vi "Draw Tree.vi"(11 "picture":refnum<vi>) -> (3 "2D Picture":picture)   [LabVIEW 2025]
uses:
  <vilib>/picture/picture.llb/imagedata.ctl
  Types/Single Cmd Info.ctl
  Types/Sequencing Tree Node.ctl
  <vilib>/Analysis/NI_AALBase.lvlib
  <vilib>/Analysis/baseanly.llb/Mean (DBL).vi
panel:
  in  "Command Height":dbl=42.0
  in  "Path on Command Branch Height":dbl=53.0
  in  "Default Path Height":dbl=25.0
  in  "Leaf Height":dbl=10.0
  in  "Leaf Circle Radius":i16
  in  "pen":T1={"Width"=3, "Style"=enum."Solid"}
  in  "2D Picture":picture
  in  "Column Gap":dbl=30.0
  in  "Line Thickness":dbl=3.0 format="%#_13g"
  in  "[user-specified font]":T2={"Font Name:"="Bahnschrift", "Size"=15, "Strikeout?"=FALSE, "Italic?"=FALSE, "Underline?"=FALSE, "Outline?"=FALSE, "Shadow?"=FALSE, "Bold?"=FALSE}
  in  "Width Padding":dbl=5.0 format="%#_13g"
  in  "Row Gap":dbl=30.0
  in  "Sequencing Data":T3[](array[typedef])
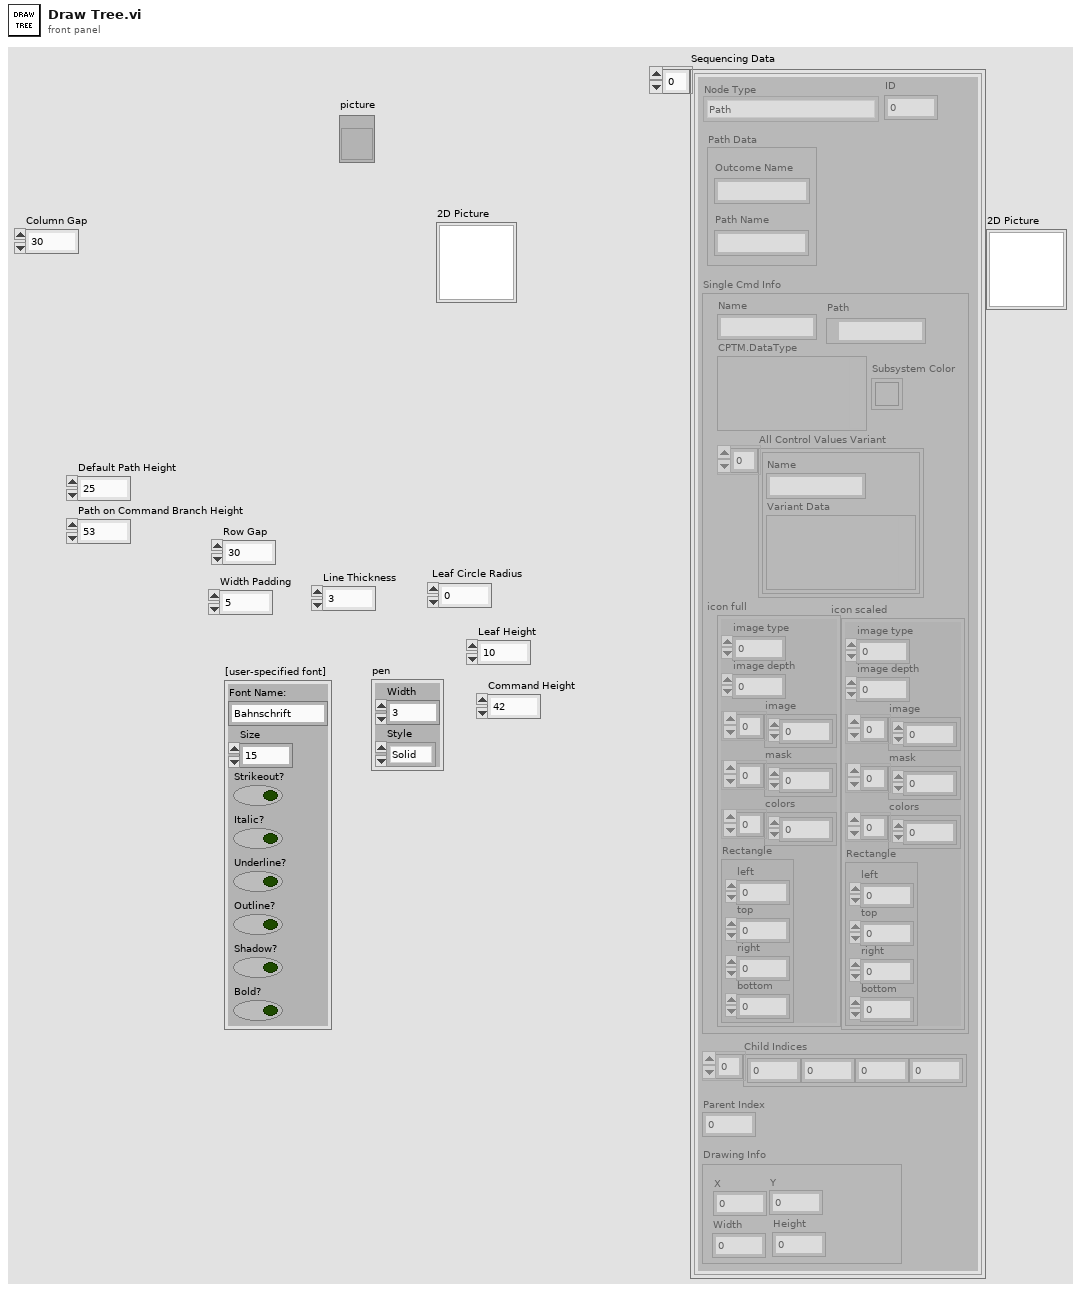
[diagram p1: front panel]
types:
  T1 = cluster{"Width":i16, "Style":enum32{"Solid", "Dash", "Dot", "DashDot", "DashDotDot"}}
  T2 = cluster{"Font Name:":string, "Size":i16, "Strikeout?":bool, "Italic?":bool, "Underline?":bool, "Outline?":bool, "Shadow?":bool, "Bold?":bool}
  T3 = typedef "Sequencing Tree Node.ctl" = cluster{"Node Type":enum16{"Path", "Command", "Leaf"}, "ID":i16, "Path Data":cluster{"Path Name":string, "Outcome Name":string}, "Single Cmd Info":T4, "Child Indices":i32[], "Parent Index":i32, "Drawing Info":cluster{"X":dbl, "Y":dbl, "Width":dbl, "Height":dbl}}
  T4 = typedef "Single Cmd Info.ctl" = cluster{"Name":string, "CPTM.DataType":variant, "All Control Values Variant":cluster{"Name":string, "Variant Data":variant}[], "icon full":T5, "icon scaled":T5, "Path":path, "Subsystem Color":u32}
  T5 = typedef "imagedata.ctl" = cluster{"image type":i32, "image depth":i32, "image":u8[], "mask":u8[], "colors":u32[], "Rectangle":cluster{"left":i16, "top":i16, "right":i16, "bottom":i16}}
  T6 = enum16{"User-specified Font", "Application Font", "System Font", "Dialog Font"}
  T7 = cluster{"Path Name":string, "Outcome Name":string}
  T8 = cluster{"X":dbl, "Y":dbl, "Width":dbl, "Height":dbl}
  T9 = cluster{"left":i16, "top":i16, "right":i16, "bottom":i16}
  T10 = cluster{"[0]":dbl, "[1]":dbl, "[2]":dbl, "[3]":dbl}
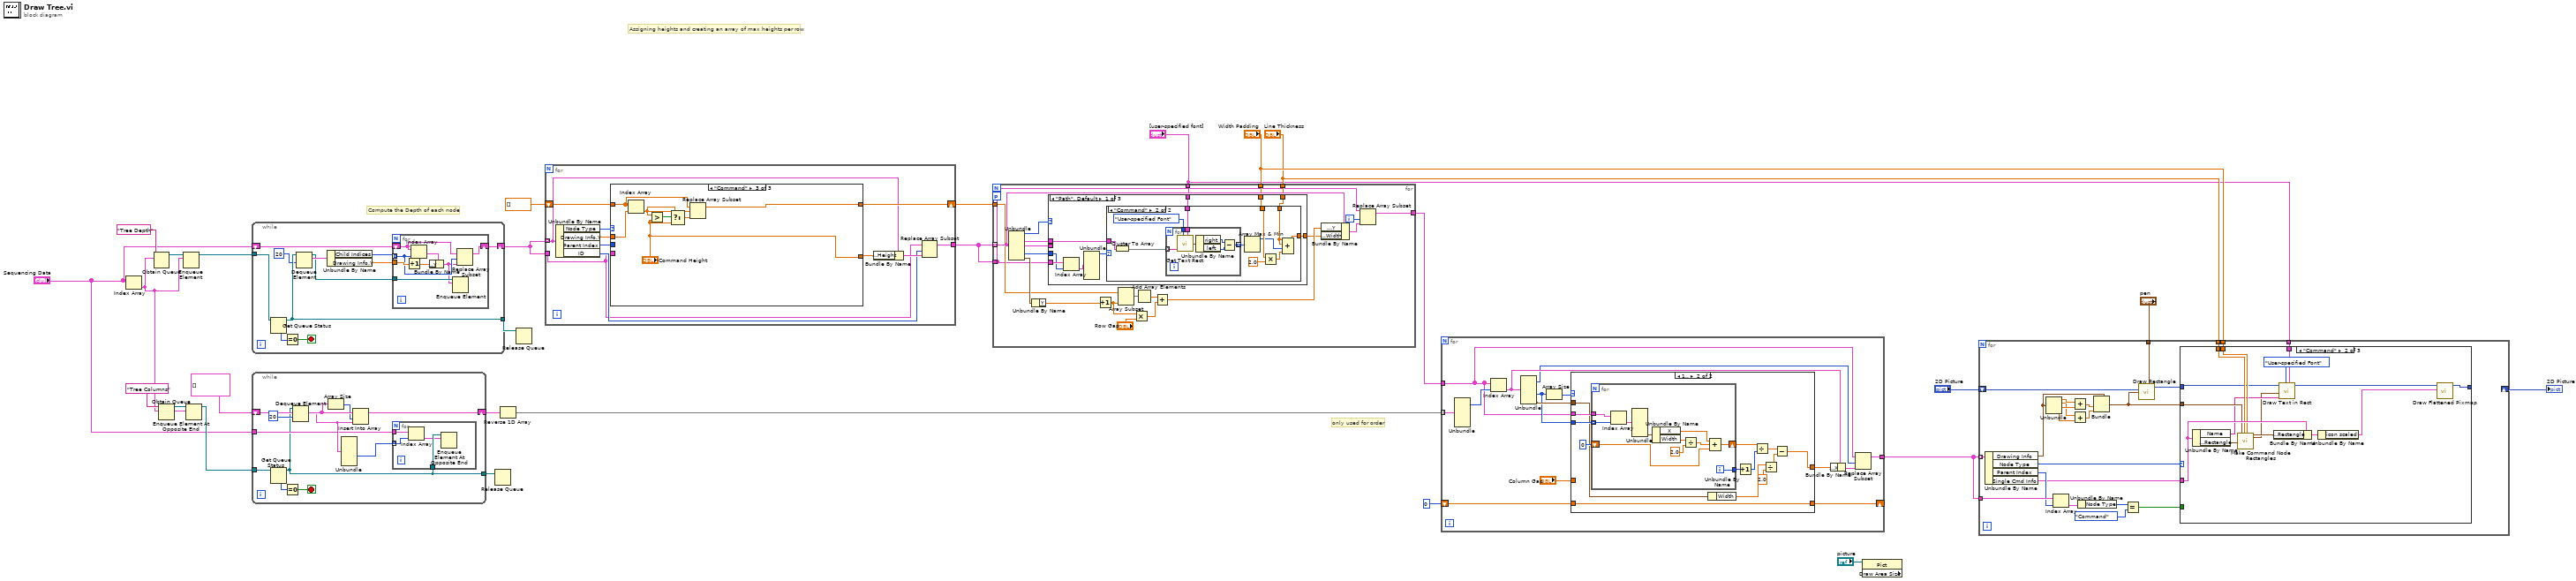
[diagram p0: block diagram]
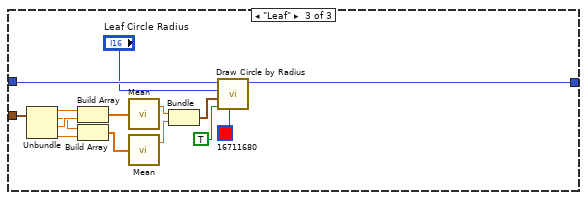
[diagram p3: hidden frame]
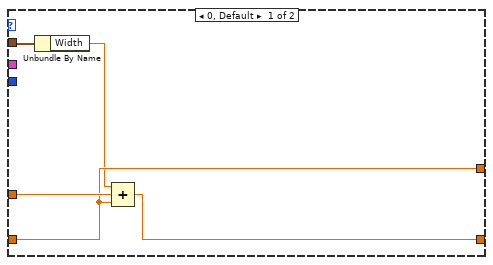
[diagram p4: hidden frame]
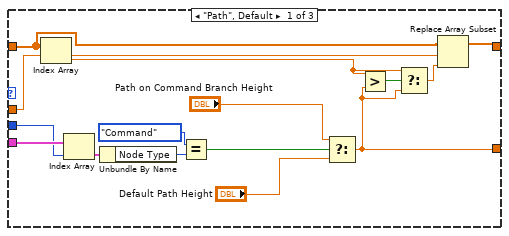
[diagram p5: hidden frame]
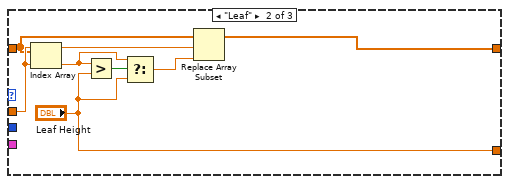
[diagram p6: hidden frame]
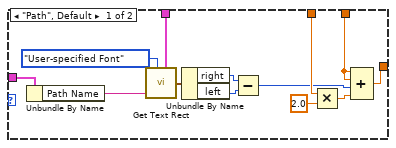
[diagram p7: hidden frame]
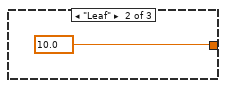
[diagram p8: hidden frame]
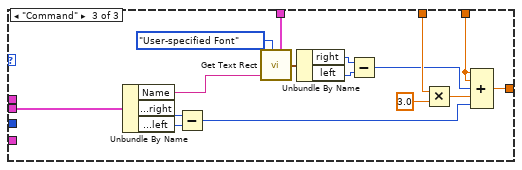
[diagram p9: hidden frame]
diagram:
  # "only used for order"
  # "Assigning heights and creating an array of max heights per row"
  # "Compute the Depth of each node"
  n1 = Index Array(array="Sequencing Data") -> (element=w19:T3)  [unwired: 1 in]
  n2 = Obtain Queue(name (unnamed)="Tree Depth", element data type=w19) -> (queue out=w25:refnum<queue>)  [unwired: 3 in, 2 out]
  n3 = Obtain Queue(name (unnamed)="Tree Columns", element data type=w19) -> (queue out=w21:refnum<queue>)  [unwired: 3 in, 2 out]
  n4 = Enqueue Element(queue=w25, element=w19) -> (queue out=w24:refnum<queue>)  [unwired: 2 in, 2 out]
  n5 = Enqueue Element At Opposite End(queue=w21, element=w19) -> (queue out=w20:refnum<queue>)  [unwired: 2 in, 2 out]
  n6 = while {
    tunnel: w24 -> [w32]
    shift-right: [w34] -> w13
    shift-left: "Sequencing Data" -> [w35]
    tunnel: [w30] -> w22
    stop <- w38 stop-if-true
    n7 = Get Queue Status(queue=w32) -> (queue out=w30:refnum<queue>, # elements in queue=w33:i32)  [unwired: 2 in, 6 out]
    n8 = Equal To 0?(x=w33) -> (x = 0?=w38:bool)
    n9 = Dequeue Element(queue=w30, timeout in ms (-1)=20) -> (queue out=w31:refnum<queue>, element=w37:T3)  [unwired: 1 in, 2 out]
    n10 = Unbundle By Name(w37) -> ("Child Indices"=w36:i32[], "Drawing Info.Y"=w28:dbl)
    n11 = for {
      tunnel: w36 -> [w43] mode=indexing
      tunnel: w28 -> [w46]
      shift-right: [w42] -> w34
      shift-left: w35 -> [w44]
      tunnel: w31 -> [w41]
      n12 = Increment(x=w46) -> (x+1=w39:dbl)
      n13 = Index Array(array=w44, index=w43) -> (element=w45:T3)
      n14 = Bundle By Name(cluster=w45, "Drawing Info.Y"=w39) -> (w40:T3)
      n15 = Enqueue Element(queue=w41, element=w40) -> ()  [unwired: 2 in, 3 out]
      n16 = Replace Array Subset(array=w44, new element=w40, index=w43) -> (w42:T3[])
    }
  }
  n17 = while {
    tunnel: [w48] -> w18
    shift-right: [w51] -> w17
    shift-left: T3[] [] ("Sequencing Data 2") -> [w53]
    tunnel: w20 -> [w55]
    tunnel: "Sequencing Data" -> [w49]
    stop <- w57 stop-if-true
    n18 = Get Queue Status(queue=w55) -> (queue out=w48:refnum<queue>, # elements in queue=w56:i32)  [unwired: 2 in, 6 out]
    n19 = Equal To 0?(x=w56) -> (x = 0?=w57:bool)
    n20 = Dequeue Element(queue=w48, timeout in ms (-1)=20) -> (element=w50:T3)  [unwired: 1 in, 3 out]
    n21 = Array Size(array=w53) -> (size(s)=w52:i32)
    n22 = Unbundle(w50) -> ("Child Indices"=w47:i32[])  [unwired: 6 out]
    n23 = Insert Into Array(array=w53, index=w52, new element=w50) -> (w51:T3[])
    n24 = for {
      tunnel: w47 -> [w60] mode=indexing
      tunnel: w49 -> [w61]
      tunnel: w48 -> [w59]
      n25 = Index Array(array=w61, index=w60) -> (element=w58:T3)
      n26 = Enqueue Element At Opposite End(queue=w59, element=w58) -> ()  [unwired: 2 in, 3 out]
    }
  }
  n27 = Release Queue(queue=w18) -> ()  [unwired: 2 in, 3 out]
  n28 = Reverse 1D Array(array=w17) -> (reversed array=w10:T3[])
  n29 = Release Queue(queue=w22) -> ()  [unwired: 2 in, 3 out]
  n30 = for {
    tunnel: w13 -> [w67] mode=indexing
    shift-right: [w69] -> w12
    shift-left: dbl[] [] -> [w70]
    tunnel: w13 -> [w63]
    tunnel: [w62] -> w11
    n31 = Unbundle By Name(w67) -> ("Node Type"=w72:enum16{"Path", "Command", "Leaf"}, "Drawing Info.Y"=w71:dbl, "Parent Index"=w68:i32, "ID"=w64:i16)
    n32 = case shown="\"Command\"" w72 {
      tunnel: w71 -> [w80 w91 w98]
      tunnel: w70 -> [w81 w90 w97]
      tunnel: [w79 w89 w96] -> w69
      tunnel: w63 -> [w87 _ _]
      tunnel: w68 -> [w86 _ _]
      tunnel: [w77 "Leaf Height" "Command Height"] -> w66
      frame "Path", Default {
        n33 = Index Array(array=w81, index=w80) -> (element=w83:dbl)
        n34 = Index Array(array=w87, index=w86) -> (element=w76:T3)
        n35 = Unbundle By Name(w76) -> ("Node Type"=w75:enum16{"Path", "Command", "Leaf"})
        n36 = Equal?(x=enum16{"Path", "Command", "Leaf"}."Command", y=w75) -> (x = y?=w85:bool)
        n37 = Select(t="Path on Command Branch Height", s=w85, f="Default Path Height") -> (s? t:f=w77:dbl)
        n38 = Greater?(x=w83, y=w77) -> (0:w84:bool)
        n39 = Select(t=w83, s=w84, f=w77) -> (s? t:f=w82:dbl)
        n40 = Replace Array Subset(array=w81, new element=w82, index=w80) -> (w79:dbl[])
      }
      frame "Leaf" {
        n41 = Index Array(array=w90, index=w91) -> (element=w93:dbl)
        n42 = Greater?(x=w93, y="Leaf Height") -> (0:w94:bool)
        n43 = Select(t=w93, s=w94, f="Leaf Height") -> (s? t:f=w92:dbl)
        n44 = Replace Array Subset(array=w90, new element=w92, index=w91) -> (w89:dbl[])
      }
      frame "Command" {
        n45 = Index Array(array=w97, index=w98) -> (element=w100:dbl)
        n46 = Greater?(x=w100, y="Command Height") -> (0:w101:bool)
        n47 = Select(t=w100, s=w101, f="Command Height") -> (s? t:f=w99:dbl)
        n48 = Replace Array Subset(array=w97, new element=w99, index=w98) -> (w96:dbl[])
      }
    }
    n49 = Bundle By Name(cluster=w67, "Drawing Info.Height"=w66) -> (w65:T3)
    n50 = Replace Array Subset(array=w63, new element=w65, index=w64) -> (w62:T3[])
  }
  n51 = for {
    tunnel: w11 -> [w122] mode=indexing
    tunnel: w12 -> [w120]
    workers-P: _ -> [_]
    tunnel: "Width Padding" -> [w111]
    tunnel: "[user-specified font]" -> [w110]
    tunnel: "Line Thickness" -> [w108]
    tunnel: w11 -> [w105]
    tunnel: [w102] -> w9
    i -> [w104]
    n52 = Unbundle(w122) -> ("Node Type"=w123:enum16{"Path", "Command", "Leaf"}, "Path Data"=w106:T7, "Single Cmd Info"=w112:T4, "Parent Index"=w107:i32, "Drawing Info"=w121:T8)  [unwired: 2 out]
    n53 = Unbundle By Name(w121) -> ("Y"=w117:dbl)
    n54 = case shown="\"Path\", Default" w123 {
      tunnel: w112 -> [_ _ w180]
      tunnel: w111 -> [w128 _ w176]
      tunnel: w110 -> [w127 _ w175]
      tunnel: [w124 w164 w169] -> w109
      tunnel: w108 -> [w126 _ w165]
      tunnel: w105 -> [w132 _ _]
      tunnel: w107 -> [w131 _ _]
      tunnel: w106 -> [w125 _ _]
      frame "Path", Default {
        n55 = Index Array(array=w132, index=w131) -> (element=w130:T3)
        n56 = Unbundle(w130) -> ("Node Type"=w129:enum16{"Path", "Command", "Leaf"})  [unwired: 6 out]
        n57 = case shown="\"Command\"" w129 {
          tunnel: w128 -> [w140 w153]
          tunnel: w127 -> [w139 w152]
          tunnel: w126 -> [w136 w151]
          tunnel: w125 -> [w138 w150]
          tunnel: [w133 w146] -> w124
          frame "Path", Default {
            n58 = Unbundle By Name(w138) -> ("Path Name"=w137:string)
            n59 = call <vilib>:"Get Text Rect.vi"("desired font(Application)"=T6."User-specified Font", "text"=w137, "[user-specified font]"=w139) -> ("rect"=w143:T9)  [unwired: 6 in]
            n60 = Unbundle By Name(w143) -> ("right"=w142:i16, "left"=w141:i16)
            n61 = Subtract(x=w142, y=w141) -> (x-y=w135:i16)
            n62 = Multiply(x=w140, y=2.0) -> (x*y=w134:dbl)
            n63 = Compound Arithmetic op=ADD(w136, w136, w135, w134) -> (w133:dbl)
          }
          frame "Command" {
            n64 = Cluster To Array(cluster=w150) -> (array=w149:string[])
            n65 = for {
              tunnel: T6."User-specified Font" ("desired font(Application)") -> [w163]
              tunnel: [w159] -> w148 mode=indexing
              tunnel: w152 -> [w158]
              tunnel: w149 -> [w157] mode=indexing
              n66 = call <vilib>:"Get Text Rect.vi"("desired font(Application)"=w163, "text"=w157, "[user-specified font]"=w158) -> ("rect"=w162:T9)  [unwired: 6 in]
              n67 = Unbundle By Name(w162) -> ("right"=w161:i16, "left"=w160:i16)
              n68 = Subtract(x=w161, y=w160) -> (x-y=w159:i16)
            }
            n69 = Array Max & Min(array=w148) -> (max value=w147:i16)  [unwired: 3 out]
            n70 = Multiply(x=w153, y=2.0) -> (x*y=w154:dbl)
            n71 = Compound Arithmetic op=ADD(w151, w151, w147, w154) -> (w146:dbl)
          }
        }
      }
      frame "Leaf" {
        w164 = 10.0 items=["Leaf"=10.0, "Default Path"=25.0, "Command"=42.0, "Path on Command Branch"=53.0] ("Height")
      }
      frame "Command" {
        n72 = Unbundle By Name(w180) -> ("Name"=w173:string, "icon scaled.Rectangle.right"=w179:i16, "icon scaled.Rectangle.left"=w178:i16)
        n73 = Subtract(x=w179, y=w178) -> (x-y=w168:i16)
        n74 = call <vilib>:"Get Text Rect.vi"("desired font(Application)"=T6."User-specified Font", "text"=w173, "[user-specified font]"=w175) -> ("rect"=w172:T9)  [unwired: 6 in]
        n75 = Unbundle By Name(w172) -> ("right"=w171:i16, "left"=w170:i16)
        n76 = Subtract(x=w171, y=w170) -> (x-y=w166:i16)
        n77 = Multiply(x=w176, y=3.0) -> (x*y=w167:dbl)
        n78 = Compound Arithmetic op=ADD(w165, w165, w166, w167, w168) -> (w169:dbl)
      }
    }
    n79 = Increment(x=w117) -> (x+1=w116:dbl)
    n80 = Array Subset(array=w120, length=w116) -> (w119:dbl[])  [unwired: 1 in]
    n81 = Multiply(x=w116, y="Row Gap") -> (x*y=w114:dbl)
    n82 = Add Array Elements(numeric array=w119) -> (sum=w118:dbl)
    n83 = Add(x=w118, y=w114) -> (x+y=w113:dbl)
    n84 = Bundle By Name(cluster=w122, "Drawing Info.Y"=w113, "Drawing Info.Width"=w109) -> (w103:T3)
    n85 = Replace Array Subset(array=w105, new element=w103, index=w104) -> (w102:T3[])
  }
  n86 = for {
    tunnel: w10 -> [w194] mode=indexing
    tunnel: w9 -> [w183]
    shift-right: [w186] -> _
    shift-left: 0 -> [w191]
    tunnel: [w181] -> w4
    n87 = Unbundle(w194) -> ("ID"=w193:i16)  [unwired: 6 out]
    n88 = Index Array(array=w183, index=w193) -> (element=w190:T3)
    n89 = Unbundle(w190) -> ("ID"=w182:i16, "Child Indices"=w185:i32[], "Drawing Info"=w187:T8)  [unwired: 4 out]
    n90 = Array Size(array=w185) -> (size(s)=w192:i32)
    n91 = case shown="1.." w192 {
      tunnel: w191 -> [w196 w212]
      tunnel: [w196 w200] -> w189
      tunnel: "Column Gap" -> [w197 _]
      tunnel: w187 -> [w199 w202]
      tunnel: [w198 w212] -> w186
      tunnel: w185 -> [_ w211]
      tunnel: w183 -> [_ w210]
      frame 0, Default {
        n92 = Unbundle By Name(w199) -> ("Width"=w195:dbl)
        n93 = Compound Arithmetic op=ADD(w195, w197, w196) -> (w198:dbl)
      }
      frame 1.. {
        n94 = for {
          tunnel: w211 -> [w223] mode=indexing
          tunnel: w210 -> [w222]
          shift-right: [w214] -> w208
          shift-left: 0 -> [w215]
          tunnel: [w213] -> w207
          i -> [w213]
          n95 = Index Array(array=w222, index=w223) -> (element=w221:T3)
          n96 = Unbundle(w221) -> ("Drawing Info"=w220:T8)  [unwired: 6 out]
          n97 = Unbundle By Name(w220) -> ("X"=w217:dbl, "Width"=w219:dbl)
          n98 = Divide(x=w219, y=2.0) -> (x/y=w216:dbl)
          n99 = Compound Arithmetic op=ADD(w217, w216, w215) -> (w214:dbl)
        }
        n100 = Unbundle By Name(w202) -> ("Width"=w201:dbl)
        n101 = Increment(x=w207) -> (x+1=w206:i32)
        n102 = Divide(x=w208, y=w206) -> (x/y=w205:dbl)
        n103 = Divide(x=w201, y=2.0) -> (x/y=w204:dbl)
        n104 = Subtract(x=w205, y=w204) -> (x-y=w200:dbl)
      }
    }
    n105 = Bundle By Name(cluster=w190, "Drawing Info.X"=w189) -> (w184:T3)
    n106 = Replace Array Subset(array=w183, new element=w184, index=w182) -> (w181:T3[])
  }
  n107 = property class="Pict" props=["Draw Area Size"](reference="picture") -> ()  [unwired: 1 in, 3 out]
  n108 = for {
    tunnel: w4 -> [w246] mode=indexing
    shift-right: [_] -> w6
    shift-left: "2D Picture" -> [w245]
    tunnel: "pen" -> [w243]
    tunnel: w4 -> [w235]
    tunnel: "Width Padding" -> [w227]
    tunnel: "Line Thickness" -> [w226]
    tunnel: "[user-specified font]" -> [w225]
    n109 = Unbundle By Name(w246) -> ("Drawing Info"=w244:T8, "Node Type"=w236:enum16{"Path", "Command", "Leaf"}, "Parent Index"=w234:i32, "Single Cmd Info"=w228:T4)
    n110 = Unbundle(w244) -> ("X"=w242:dbl, "Y"=w240:dbl, "Width"=w241:dbl, "Height"=w239:dbl)
    n111 = Index Array(array=w235, index=w234) -> (element=w233:T3)
    n112 = Add(x=w242, y=w241) -> (x+y=w238:dbl)
    n113 = Add(x=w240, y=w239) -> (x+y=w237:dbl)
    n114 = Unbundle By Name(w233) -> ("Node Type"=w232:enum16{"Path", "Command", "Leaf"})
    n115 = Bundle(cluster=w244, "Width"=w238, "Height"=w237) -> (w229:T8)  [unwired: 2 in]
    n116 = Equal?(x=w232, y=enum16{"Path", "Command", "Leaf"}."Command") -> (x = y?=w224:bool)
    n117 = call <vilib>:"Draw Rectangle.vi"("picture"=w245, "rect"=w229, "pen"=w243) -> ("new picture"=w230:picture)  [unwired: 6 in]
    n118 = case shown="\"Command\"" w236 {
      tunnel: w230 -> [_ w249 w276]
      tunnel: w229 -> [_ w254 w274]
      tunnel: [_ w247 w262] -> _
      tunnel: w228 -> [_ w256 _]
      tunnel: w227 -> [_ w253 _]
      tunnel: w226 -> [_ w252 _]
      tunnel: w225 -> [_ w258 _]
      tunnel: w224 -> [_ _ _]
      frame "Path", Default {
      }
      frame "Command" {
        n119 = Unbundle By Name(w256) -> ("Name"=w251:string, "icon scaled.Rectangle"=w255:T9)
        n120 = call "Make Command Node Rectangles.vi"("Icon Rectangle"=w255, "Node Rectangle"=w254, "Line Thickness"=w252, "Width Padding"=w253) -> ("New Icon Rectangle"=w261:T10, "Text Rectangle"=w250:T10)  [unwired: 14 in]
        n121 = Bundle By Name(cluster=w256, "icon scaled.Rectangle"=w261) -> (w260:T4)
        n122 = call <vilib>:"Draw Text in Rect.vi"("[user-specified font]"=w258, "desired font(Application)"=T6."User-specified Font", "text"=w251, "rect"=w250, "picture"=w249) -> ("new picture"=w248:picture)  [unwired: 6 in]
        n123 = Unbundle By Name(w260) -> ("icon scaled"=w259:T5)
        n124 = call <vilib>:"Draw Flattened Pixmap.vi"("image data"=w259, "picture"=w248) -> ("new picture"=w247:picture)  [unwired: 7 in]
      }
      frame "Leaf" {
        n125 = Unbundle(w274) -> ("X"=w273:dbl, "Y"=w271:dbl, "Width"=w272:dbl, "Height"=w270:dbl)
        n126 = Build Array(w273, w272) -> (w269:dbl[])
        n127 = Build Array(w271, w270) -> (w268:dbl[])
        n128 = call-poly <vilib>:"Mean.vi"("X"=w269) -> ("mean"=w267:dbl)  [unwired: 1 out]
        n129 = call-poly <vilib>:"Mean.vi"("X"=w268) -> ("mean"=w266:dbl)  [unwired: 1 out]
        n130 = Bundle("mean"=w267, "mean"=w266) -> (w265:cluster{"mean":dbl, "mean":dbl})  [unwired: 1 in]
        n131 = call <vilib>:"Draw Circle by Radius.vi"("color(black)"=u32 16711680, "fill?(F)"=TRUE, "pixel center"=w265, "radius"="Leaf Circle Radius", "picture"=w276) -> ("new picture"=w262:picture)  [unwired: 6 in]
      }
    }
  }
  "2D Picture" <- w6
